vi "test Get-Set Terminal Name.vi"(8 "error in":errorcluster, 11 "TestCase in":refnum<class "Scripting.lvclass">) -> (0 "error out":errorcluster, 3 "TestCase out":refnum<class "Scripting.lvclass">)   [LabVIEW 2020, in "Scripting.lvclass"]
uses:
  Scripting.lvclass
  C:/dev/git/niveristand-custom-device-testing-tools/VeriStandScriptingTestCase/VeriStandScriptingTestCase.lvclass
  Shared/Address.ctl
  niveristand-custom-device-testing-tools/VeriStandScriptingTestCase/VeriStandScriptingTestCase.lvclass/VeriStandScriptingTestCase.ctl
  niveristand-custom-device-testing-tools/VeriStandScriptingTestCase/Read Target.vi
  NationalInstruments.VeriStand.SystemDefinitionAPI
  <vilib>/addons/_JKI Toolkits/VI Tester/TestCase.llb/TestCase.lvclass
  Scripting/AIM MIL-STD-1553 Scripting.lvlib
  C:/Program Files (x86)/National Instruments/LabVIEW 2020/vi.lib/addons/_JKI Toolkits/VI Tester/TestCase.llb/TestCase.lvclass
  C:/dev/git/niveristand-aim-milStd1553-custom-device/Source/Custom Device Support/Tests/Unit/Scripting/Scripting.lvclass
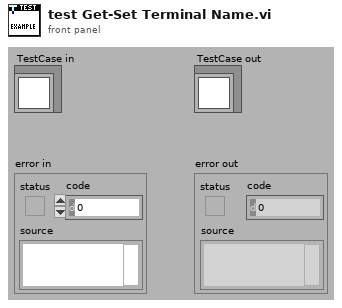
[diagram p1: front panel]
types:
  T1 = typedef "Address.ctl" = u16
  T2 = typedef "Custom Device API.lvlib/Custom Device Item Ref.ctl" = u64
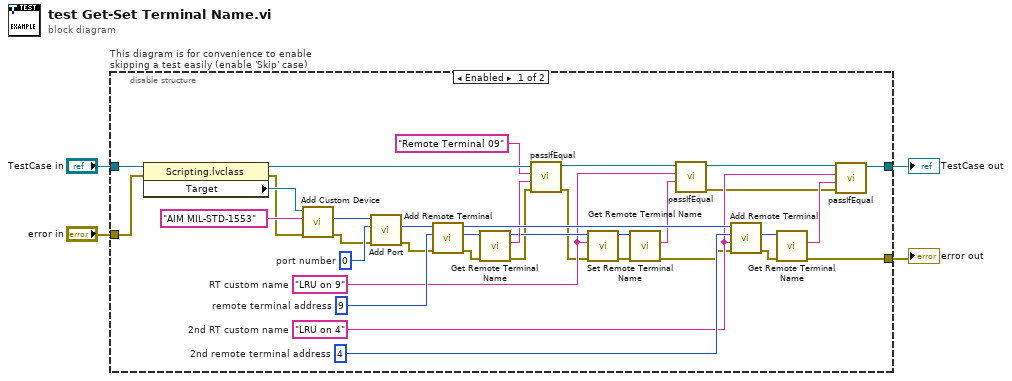
[diagram p0: block diagram]
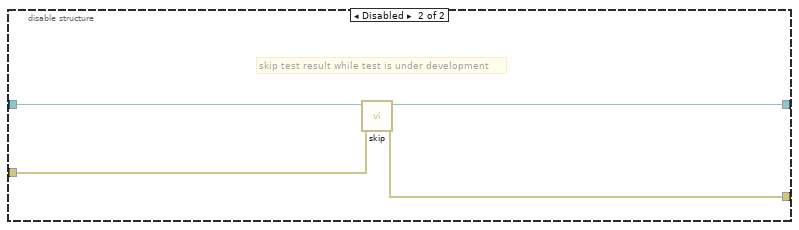
[diagram p2: hidden frame]
diagram:
  n1 = disable-structure "This diagram is for convenience to enable skipping a test easily (enable 'Skip' case)" shown="Enabled" {
    disable-tunnel: "TestCase in" -> [w38 w43]
    disable-tunnel: [w18 w41] -> w1
    disable-tunnel: [w28 w42] -> w3
    disable-tunnel: "error in" -> [w29 w40]
    frame Enabled {
      w11 = "LRU on 9"  # RT custom name
      w21 = "LRU on 4"  # 2nd RT custom name
      w27 = T1 4  # 2nd remote terminal address
      w35 = T1 9  # remote terminal address
      w36 = u16 0  # port number
      n2 = property class="Scripting.lvclass"(reference=w38, error in=w29) -> (reference out=w34:refnum<class "Scripting.lvclass">, error out=w10:errorcluster, "Target"=w37:refnum<k24>)
      n3 = call "Add Custom Device.vi"("error in"=w10, "custom device name"="AIM MIL-STD-1553" ("name"), "target"=w37) -> ("error out"=w32:errorcluster, "custom device ref out"=w33:T2)  [unwired: 6 in, 1 out]
      n4 = call "Add Port.vi"("error in"=w32, "port number"=w36, "custom device ref"=w33) -> ("error out"=w9:errorcluster, "port"=w31:T2)  [unwired: 6 in, 1 out]
      n5 = call "Add Remote Terminal.vi"("error in"=w9, "terminal address"=w35, "port"=w31) -> ("error out"=w7:errorcluster, "remote terminal"=w8:T2, "port out"=w30:T2)  [unwired: 6 in]
      n6 = call "Get Remote Terminal Name.vi"("error in"=w7, "remote terminal"=w8) -> ("error out"=w6:errorcluster, "terminal name"=w26:string, "remote terminal out"=w17:T2)  [unwired: 7 in]
      n7 = call-dynamic "passIfEqual.vi"("error in (no error)"=w6, "y"=w26, "x"="Remote Terminal 09" ("terminal name"), "TestCase in"=w34) -> ("error out"=w5:errorcluster, "TestCase out"=w16:refnum<class "Scripting.lvclass">)  [unwired: 6 in]
      n8 = call "Set Remote Terminal Name.vi"("error in"=w5, "terminal name"=w11, "remote terminal"=w17) -> ("error out"=w14:errorcluster, "remote terminal out"=w15:T2)  [unwired: 7 in]
      n9 = call "Get Remote Terminal Name.vi"("error in"=w14, "remote terminal"=w15) -> ("error out"=w13:errorcluster, "terminal name"=w12:string)  [unwired: 7 in, 1 out]
      n10 = call-dynamic "passIfEqual.vi"("y"=w12, "x"=w11, "TestCase in"=w16) -> ("error out"=w19:errorcluster, "TestCase out"=w20:refnum<class "Scripting.lvclass">)  [unwired: 7 in]
      n11 = call "Add Remote Terminal.vi"("error in"=w13, "terminal name"=w21, "terminal address"=w27, "port"=w30) -> ("error out"=w23:errorcluster, "remote terminal"=w24:T2)  [unwired: 5 in, 1 out]
      n12 = call "Get Remote Terminal Name.vi"("error in"=w23, "remote terminal"=w24) -> ("error out"=w28:errorcluster, "terminal name"=w22:string)  [unwired: 7 in, 1 out]
      n13 = call-dynamic "passIfEqual.vi"("error in (no error)"=w19, "y"=w22, "x"=w21, "TestCase in"=w20) -> ("TestCase out"=w18:refnum<class "Scripting.lvclass">)  [unwired: 6 in, 1 out]
    }
    frame Disabled {
      # "skip test result while test is under development"
      n14 = call <vilib>:"skip.vi"("error in (no error)"=w40, "TestCase in"=w43) -> ("error out"=w42:errorcluster, "TestCase out"=w41:refnum<class "Scripting.lvclass">)  [unwired: 8 in]
    }
  }
  "error out" <- w3
  "TestCase out" <- w1
